vi "gearGrabber.vi"(8 "error in (no error)":errorcluster, 9 "gear":string="My Servo RefNum", 11 "xbox":string="My Joystick RefNum") -> (0 "error out":errorcluster)   [LabVIEW 2016]
uses:
  <vilib>/Rock Robotics/WPI/Utilities/WPI_GetSetVariantRefNum.vi
  gearValue.vi
  External.lvlib
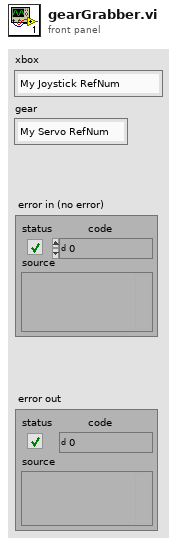
[diagram p1: front panel]
types:
  T1 = typedef "WPI_JoystickDevRef.ctl" = cluster{"Device":T2}
  T2 = typedef "WPI_JoystickDeviceEnum.ctl" = enum16{"USB 0", "USB 1", "USB 2", "USB 3", "USB 4", "USB 5"}
  T3 = typedef "WPI_ServoDeviceRef.ctl" = cluster{"DeviceStatus":errorcluster, "PWM Channel":T4, "DeadBand":T5}
  T4 = typedef "FPGA_DIOPWMChannel.ctl" = enum8{"PWM 0", "PWM 1", "PWM 2", "PWM 3", "PWM 4", "PWM 5", "PWM 6", "PWM 7", "PWM 8", "PWM 9", "PWM MXP 0", "PWM MXP 1", "PWM MXP 2", "PWM MXP 3", "PWM MXP 4", "PWM MXP 5", "PWM MXP 6", "PWM MXP 7", "PWM MXP 8", "PWM MXP 9", "Invalid"}
  T5 = typedef "WPI_PWMDeadband.ctl" = cluster{"Name":string, "maxPositivePwm":i32, "minPositivePwm":i32, "centerPwm":i32, "maxNegativePwm":i32, "minNegativePwm":i32, "angularRange":u16}
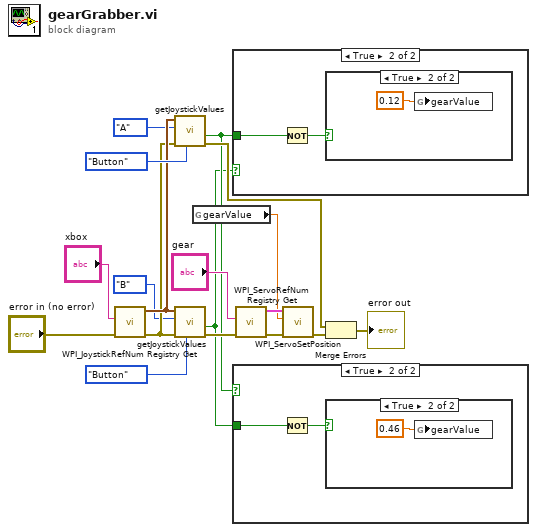
[diagram p0: block diagram]
diagram:
  n1 = call <vilib>:"WPI_JoystickRefNum Registry Get.vi"("error in (no error)"="error in (no error)", "refnum name"="xbox") -> ("error out"=w15:errorcluster, "JoystickDevRef"=w16:T1)  [unwired: 8 in]
  n2 = call "getJoystickValues.vi"("Mode"=enum16{"Axis", "Button"}."Button", "error in (no error)"=w15, "buttonType"=enum16{"A", "B", "X", "Y", "LB", "RB"}."A", "JoystickDevRef"=w16) -> ("error out"=w9:errorcluster, "Button Pressed"=w2:bool)  [unwired: 4 in, 2 out]
  n3 = call "getJoystickValues.vi"("Mode"=enum16{"Axis", "Button"}."Button", "error in (no error)"=w15, "buttonType"=enum16{"A", "B", "X", "Y", "LB", "RB"}."B", "JoystickDevRef"=w16) -> ("error out"=w10:errorcluster, "Button Pressed"=w1:bool)  [unwired: 4 in, 2 out]
  n4 = global read "gearValue.vi" "gearValue"() -> (w12:dbl)
  n5 = case shown="True" w1 {
    tunnel: w2 -> [_ w20]
    frame False {
    }
    frame True {
      n6 = Not(x=w20) -> (.not. x?=w19:bool)
      n7 = case shown="True" w19 {
        frame False {
        }
        frame True {
          n8 = global write "gearValue.vi" "gearValue"(0.12 ("gearValue")) -> ()
        }
      }
    }
  }
  n9 = case shown="True" w2 {
    tunnel: w1 -> [_ w23]
    frame False {
    }
    frame True {
      n10 = Not(x=w23) -> (.not. x?=w22:bool)
      n11 = case shown="True" w22 {
        frame False {
        }
        frame True {
          n12 = global write "gearValue.vi" "gearValue"(0.46 ("gearValue")) -> ()
        }
      }
    }
  }
  n13 = call <vilib>:"WPI_ServoRefNum Registry Get.vi"("error in (no error)"=w10, "refnum name"="gear") -> ("error out"=w13:errorcluster, "ServoDeviceRef"=w14:T3)  [unwired: 8 in]
  n14 = call <vilib>:"WPI_ServoSetPosition.vi"("error in (no error)"=w13, "Position"=w12, "ServoDeviceRef"=w14) -> ("error out"=w6:errorcluster)  [unwired: 7 in, 1 out]
  n15 = Merge Errors(w9, w6) -> (→"error out":errorcluster)
